vi "Statistics.EWMA.vi"(5 "InitialValue":dbl format="%#_13g", 7 "Weight":dbl=0.001 min=0.0001 max=0.9999 step=0.0001 format="%#_13g", 11 "Input":dbl format="%#_13g") -> (3 "Output":dbl)   [LabVIEW 2016]
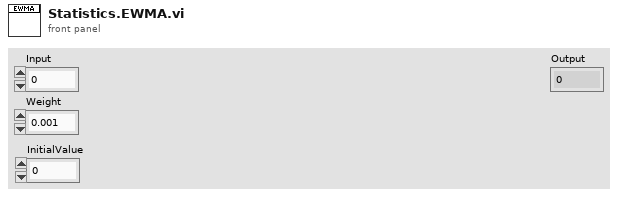
[diagram p1: front panel]
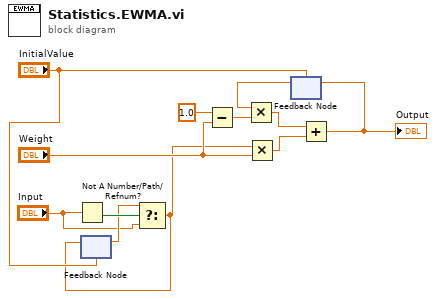
[diagram p0: block diagram]
diagram:
  n1 = Not A Number/Path/Refnum?(number/path/refnum="Input") -> (NaN/Path/Refnum?=w5:bool)
  n2 = feedback #1("InitialValue") -> (w4:dbl)
  n3 = Select(t=w4, s=w5, f="Input") -> (s? t:f=w1:dbl)
  n4 = feedback-in #1(w1) -> ()
  n5 = Subtract(x=1.0, y="Weight") -> (x-y=w10:dbl)
  n6 = Multiply(x=w1, y="Weight") -> (x*y=w8:dbl)
  n7 = feedback #2("InitialValue") -> (w6:dbl)
  n8 = Multiply(x=w6, y=w10) -> (x*y=w9:dbl)
  n9 = Add(x=w9, y=w8) -> (x+y=w7:dbl)
  "Output" <- w7
  n10 = feedback-in #2(w7) -> ()
